vi "SET_HEADING.vi"(10 "argv":string[](array[string]), 11 "args":u8) -> ()   [LabVIEW 2015]
uses:
  Team Code/Robot Global Data.vi
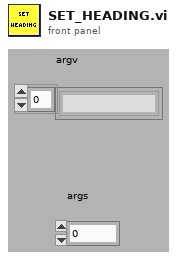
[diagram p1: front panel]
types:
  T1 = typedef "WPI_GyroDevRef.ctl" = cluster{"DevStatus":errorcluster, "Analog Channel":T2, "Offset":dbl, "Gain (VoltsPerDegree/Second)":dbl}
  T2 = typedef "FPGA_AIChannel.ctl" = enum8{"AI 0", "AI 1", "AI 2", "AI 3", "AI MXP 0", "AI MXP 1", "AI MXP 2", "AI MXP 3", "Invalid"}
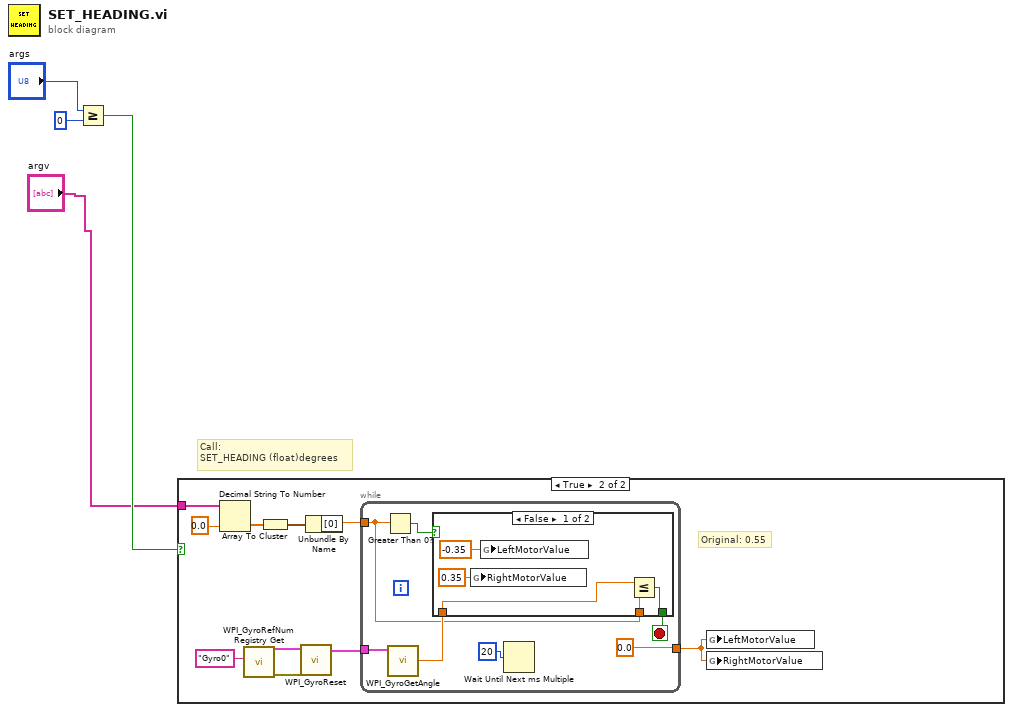
[diagram p0: block diagram]
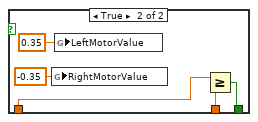
[diagram p3: hidden frame]
diagram:
  # "Call:\nSET_HEADING (float)degrees"
  n1 = Greater Or Equal?(x="args", y=u8 0) -> (x >= y?=w4:bool)
  n2 = case shown="True" w4 {
    tunnel: "argv" -> [_ w14]
    frame False {
    }
    frame True {
      # "Original: 0.55"
      n3 = Decimal String To Number(string=w14, default (0L)=0.0 ("default (0 I32)")) -> (number=w12:dbl[])  [unwired: 2 out]
      n4 = call <vilib>:"WPI_GyroRefNum Registry Get.vi"("refnum name"="Gyro0") -> ("error out"=w7:errorcluster, "GyroDevRef"=w5:T1)  [unwired: 9 in]
      n5 = Array To Cluster(array=w12) -> (cluster=w11:cluster{"[0]":dbl, "[1]":dbl})
      n6 = call <vilib>:"WPI_GyroReset.vi"("error in (no error)"=w7, "GyroDevRef"=w5) -> ("GyroDevRef"=w6:T1)  [unwired: 8 in, 1 out]
      n7 = Unbundle By Name(w11) -> ("[0]"=w10:dbl)
      n8 = while {
        tunnel: w10 -> [w15]
        tunnel: w6 -> [w19]
        tunnel: [0.0 ("LeftMotorValue")] -> w8
        stop <- w17 stop-if-true
        n9 = Greater Than 0?(x=w15) -> (x > 0?=w20:bool)
        n10 = call <vilib>:"WPI_GyroGetAngle.vi"("GyroDevRef"=w19) -> ("Angle"=w18:dbl)  [unwired: 7 in, 3 out]
        n11 = case shown="False" w20 {
          tunnel: w18 -> [w23 w28]
          tunnel: [w24 w29] -> w17
          tunnel: w15 -> [w22 w27]
          frame False {
            n12 = global write "Robot Global Data.vi" "RightMotorValue"(0.35 ("LeftMotorValue")) -> ()
            n13 = global write "Robot Global Data.vi" "LeftMotorValue"(-0.35 ("LeftMotorValue")) -> ()
            n14 = Less Or Equal?(x=w23, y=w22) -> (x <= y?=w24:bool)
          }
          frame True {
            n15 = global write "Robot Global Data.vi" "RightMotorValue"(-0.35 ("LeftMotorValue")) -> ()
            n16 = global write "Robot Global Data.vi" "LeftMotorValue"(0.35 ("LeftMotorValue")) -> ()
            n17 = Greater Or Equal?(x=w28, y=w27) -> (x >= y?=w29:bool)
          }
        }
        n18 = Wait Until Next ms Multiple(millisecond multiple=u32 20) -> ()  [unwired: 1 out]
      }
      n19 = global write "Robot Global Data.vi" "LeftMotorValue"(w8) -> ()
      n20 = global write "Robot Global Data.vi" "RightMotorValue"(w8) -> ()
    }
  }
